vi "Serve Buffers.vi"(8 "error in (no error)":errorcluster, 11 "Data Server Thread in":refnum<class "Data Server Thread.lvclass">) -> (0 "error out":errorcluster, 3 "Data Server Thread out":refnum<class "Data Server Thread.lvclass">)   [LabVIEW 2017, in "DSF Core.lvlib" / "Data Server Thread.lvclass"]
uses:
  Data Server Thread.lvclass
  Data Server Thread.lvclass/Data Server Thread.ctl
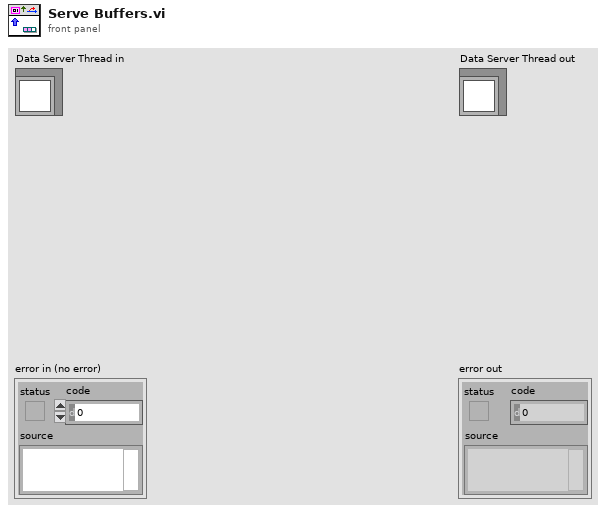
[diagram p1: front panel]
types:
  T1 = typedef "DSF Core.lvlib/Data Server Thread.lvclass/Viewer Data.ctl" = cluster{"remote address":string, "remote port":u16, "connection ID":refnum<k5>, "Buffer":refnum<class "Buffer.lvclass">}
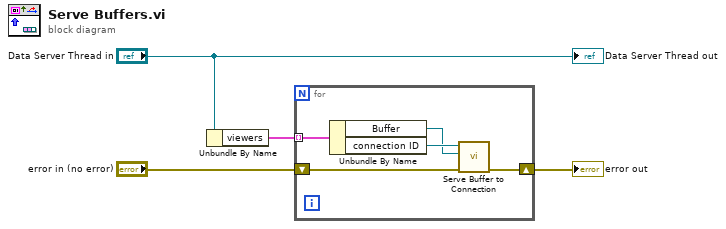
[diagram p0: block diagram]
diagram:
  n1 = Unbundle By Name("Data Server Thread in") -> ("viewers"=w3:T1[])
  n2 = for {
    tunnel: w3 -> [w8] mode=indexing
    shift-right: [w9] -> w4
    shift-left: "error in (no error)" -> [w6]
    n3 = Unbundle By Name(w8) -> ("Buffer"=w5:refnum<class "Buffer.lvclass">, "connection ID"=w7:refnum<k5>)
    n4 = call "Serve Buffer to Connection.vi"("error in (no error)"=w6, "Buffer"=w5, "connection ID in"=w7) -> ("error out"=w9:errorcluster)  [unwired: 7 in, 1 out]
  }
  "error out" <- w4
  "Data Server Thread out" <- "Data Server Thread in"
